vi "solar_voy_def LVType to Type.vi"(9 "Each Array Item (256 bits) [1D Str only]":i32=256, 10 "Variable Size (0 bits = rest)":i32, 11 "LVTYPE":T1) -> (1 "EACH_SIZE (0=NoArray)":i32, 2 "TOTAL_SIZE (0)":i32, 3 "TYPE (BLOCK)":T2)   [LabVIEW 2018]
doc: "This converts a LabVIEW data type to a COSMOS type."
uses:
  solar_voy_def_ctl ITEM TYPE.ctl
  type/solar_type Item Type.ctl
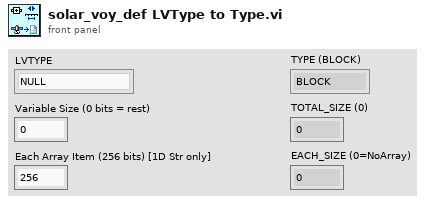
[diagram p1: front panel]
types:
  T1 = typedef "solar_type Item Type.ctl" = enum16{"NULL", "UNKNOWN", "CLUSTER", "I8", "I16", "I32", "I64", "U8", "U16", "U32", "U64", "U8_ENUM", "U16_ENUM", "U32_ENUM", "SGL", "DBL", "BOOLEAN", "STRING", "PATH", "VISA", "TAG", "TIME", "I8_1D", "I16_1D", "I32_1D", "I64_1D", "U8_1D", "U16_1D", "U32_1D", "U64_1D", "U8_ENUM_1D", "U16_ENUM_1D", "U32_ENUM_1D", "SGL_1D", "DBL_1D", "BOOLEAN_1D", "STRING_1D", "PATH_1D", "VISA_1D", "TAG_1D", "TIME_1D", "I8_2D", "I16_2D", "I32_2D", "I64_2D", "U8_2D", "U16_2D", "U32_2D", "U64_2D", "U8_ENUM_2D", "U16_ENUM_2D", "U32_ENUM_2D", "SGL_2D", "DBL_2D", "BOOLEAN_2D", "STRING_2D", "PATH_2D", "VISA_2D", "TAG_2D", "TIME_2D"}
  T2 = typedef "solar_voy_def_ctl ITEM TYPE.ctl" = enum8{"BLOCK", "INT", "UINT", "FLOAT", "STRING"}
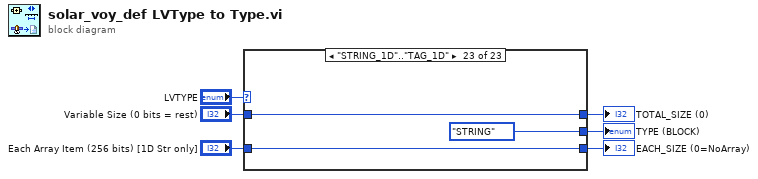
[diagram p0: block diagram]
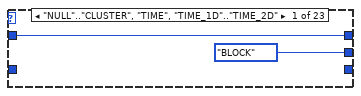
[diagram p2: hidden frame]
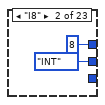
[diagram p3: hidden frame]
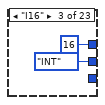
[diagram p4: hidden frame]
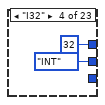
[diagram p5: hidden frame]
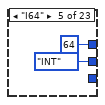
[diagram p6: hidden frame]
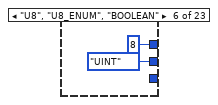
[diagram p7: hidden frame]
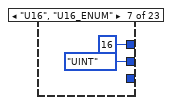
[diagram p8: hidden frame]
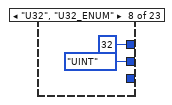
[diagram p9: hidden frame]
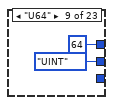
[diagram p10: hidden frame]
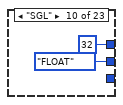
[diagram p11: hidden frame]
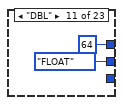
[diagram p12: hidden frame]
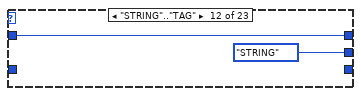
[diagram p13: hidden frame]
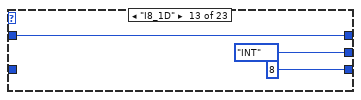
[diagram p14: hidden frame]
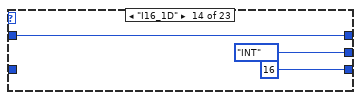
[diagram p15: hidden frame]
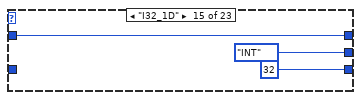
[diagram p16: hidden frame]
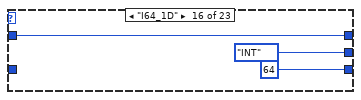
[diagram p17: hidden frame]
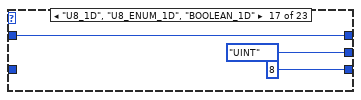
[diagram p18: hidden frame]
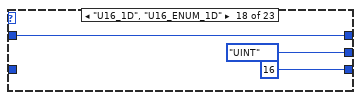
[diagram p19: hidden frame]
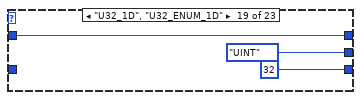
[diagram p20: hidden frame]
diagram:
  n1 = case shown="\"STRING_1D\"..\"TAG_1D\"" "LVTYPE" {
    tunnel: [w8 8 ("TOTAL_SIZE (0)") 16 ("TOTAL_SIZE (0)") 32 ("TOTAL_SIZE (0)") 64 ("TOTAL_SIZE (0)") 8 ("TOTAL_SIZE (0)") 16 ("TOTAL_SIZE (0)") 32 ("TOTAL_SIZE (0)") 64 ("TOTAL_SIZE (0)") 32 ("TOTAL_SIZE (0)") 64 ("TOTAL_SIZE (0)") w30 w32 w35 w38 w41 w44 w47 w50 w53 w56 w59 w63] -> w6
    tunnel: [solar_voy_def_ctl_ITEM_TYPE."BLOCK" ("TYPE") solar_voy_def_ctl_ITEM_TYPE."INT" ("TYPE") solar_voy_def_ctl_ITEM_TYPE."INT" ("TYPE") solar_voy_def_ctl_ITEM_TYPE."INT" ("TYPE") solar_voy_def_ctl_ITEM_TYPE."INT" ("TYPE") solar_voy_def_ctl_ITEM_TYPE."UINT" ("TYPE") solar_voy_def_ctl_ITEM_TYPE."UINT" ("TYPE") solar_voy_def_ctl_ITEM_TYPE."UINT" ("TYPE") solar_voy_def_ctl_ITEM_TYPE."UINT" ("TYPE") solar_voy_def_ctl_ITEM_TYPE."FLOAT" ("TYPE") solar_voy_def_ctl_ITEM_TYPE."FLOAT" ("TYPE") solar_voy_def_ctl_ITEM_TYPE."STRING" ("TYPE") solar_voy_def_ctl_ITEM_TYPE."INT" ("TYPE") solar_voy_def_ctl_ITEM_TYPE."INT" ("TYPE") solar_voy_def_ctl_ITEM_TYPE."INT" ("TYPE") solar_voy_def_ctl_ITEM_TYPE."INT" ("TYPE") solar_voy_def_ctl_ITEM_TYPE."UINT" ("TYPE") solar_voy_def_ctl_ITEM_TYPE."UINT" ("TYPE") solar_voy_def_ctl_ITEM_TYPE."UINT" ("TYPE") solar_voy_def_ctl_ITEM_TYPE."UINT" ("TYPE") solar_voy_def_ctl_ITEM_TYPE."FLOAT" ("TYPE") solar_voy_def_ctl_ITEM_TYPE."FLOAT" ("TYPE") solar_voy_def_ctl_ITEM_TYPE."STRING" ("TYPE")] -> w5
    tunnel: [_ _ _ _ _ _ _ _ _ _ _ _ 8 ("TOTAL_SIZE (0)") 16 ("TOTAL_SIZE (0)") 32 ("TOTAL_SIZE (0)") 64 ("TOTAL_SIZE (0)") 8 ("TOTAL_SIZE (0)") 16 ("TOTAL_SIZE (0)") 32 ("TOTAL_SIZE (0)") 64 ("TOTAL_SIZE (0)") 32 ("TOTAL_SIZE (0)") 64 ("TOTAL_SIZE (0)") w62] -> w4
    tunnel: "Variable Size (0 bits = rest)" -> [w8 _ _ _ _ _ _ _ _ _ _ w30 w32 w35 w38 w41 w44 w47 w50 w53 w56 w59 w63]
    tunnel: "Each Array Item (256 bits) [1D Str only]" -> [_ _ _ _ _ _ _ _ _ _ _ _ _ _ _ _ _ _ _ _ _ _ w62]
    frame "NULL".."CLUSTER", "TIME", "TIME_1D".."TIME_2D" {
    }
    frame "I8" {
    }
    frame "I16" {
    }
    frame "I32" {
    }
    frame "I64" {
    }
    frame "U8", "U8_ENUM", "BOOLEAN" {
    }
    frame "U16", "U16_ENUM" {
    }
    frame "U32", "U32_ENUM" {
    }
    frame "U64" {
    }
    frame "SGL" {
    }
    frame "DBL" {
    }
    frame "STRING".."TAG" {
    }
    frame "I8_1D" {
    }
    frame "I16_1D" {
    }
    frame "I32_1D" {
    }
    frame "I64_1D" {
    }
    frame "U8_1D", "U8_ENUM_1D", "BOOLEAN_1D" {
    }
    frame "U16_1D", "U16_ENUM_1D" {
    }
    frame "U32_1D", "U32_ENUM_1D" {
    }
    frame "U64_1D" {
    }
    frame "SGL_1D" {
    }
    frame "DBL_1D" {
    }
    frame "STRING_1D".."TAG_1D" {
    }
  }
  "TOTAL_SIZE (0)" <- w6
  "TYPE (BLOCK)" <- w5
  "EACH_SIZE (0=NoArray)" <- w4
